vi "test_av_array_cast.vi"() -> ()   [LabVIEW 2013]
uses:
  <vilib>/userdefined/High Color/nirio_resource_hc.ctl
  <vilib>/FPGAPlugInAG/PXIe-7975R/niLvFpga_Open_PXIe-7975R.vi
  <vilib>/rvi/interface/common/dynamic/niFpgaDynamicAddResources.vi
  <vilib>/rvi/interface/common/niFpgaWaitOnOcc.vi
  <vilib>/Utility/error.llb/Error Cluster From Error Code.vi
  <vilib>/rvi/errors/niLvFpgaAdjustHostInterfaceError.vi
  <vilib>/rvi/interface/nirviOpenFPGA/nirviOpenFPGA.xnode
  FPGA Bitfiles/mixer_FPGATarget3_arraysizetest_DYaVQgTtPqo.lvbitx
  <vilib>/rvi/interface/nirviReadWriteControl/nirviReadWriteControl.xnode
  NiFpgaLv.dll
  <vilib>/rvi/interface/Simulation/niFpgaSimulationCallBeginRW.vi
panel:
  out "error out 2":errorcluster
  out "error out":errorcluster
  in  "stop":bool
  out "array 4 to 8":fxp<+/-,16,14>[](array[numeric])
  out "array 4 out":fxp<+/-,16,14>[](array[numeric])
  in  "4 in":fxp<+/-,16,14>[](array[numeric])=[0.0, 0.0, 0.0, 0.0]
  in  "4 in":bool
  in  "8 in":bool
  in  "array 8 in":fxp<+/-,16,14>[](array[numeric])=[0.0, 0.0, 0.0, 0.0, 0.0, 0.0, 0.0, 0.0]
  out "array 8 out":fxp<+/-,16,14>[](array[numeric])
  out "array 8 to 4":fxp<+/-,16,14>[](array[numeric])
  in  "resource name":T1="RIO0"
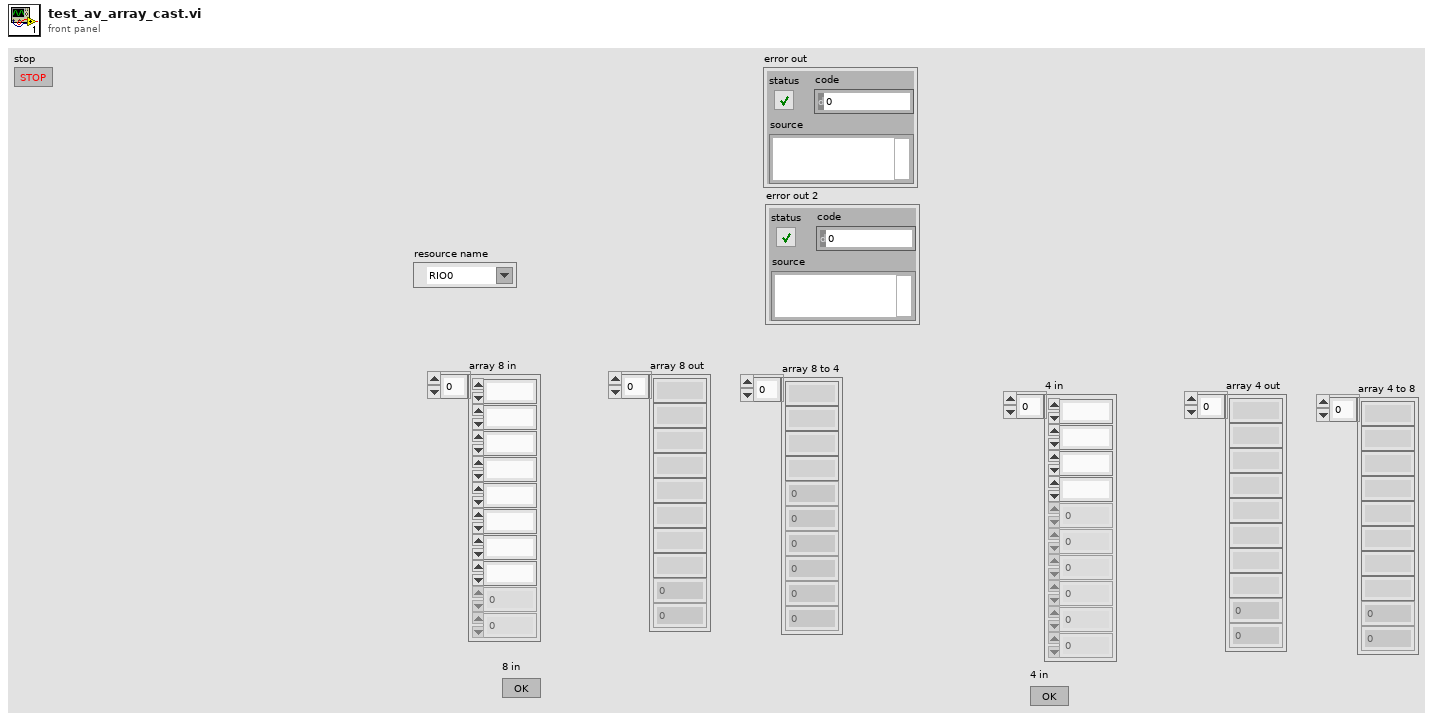
[diagram p1: front panel]
types:
  T1 = typedef "nirio_resource_hc.ctl" = tag
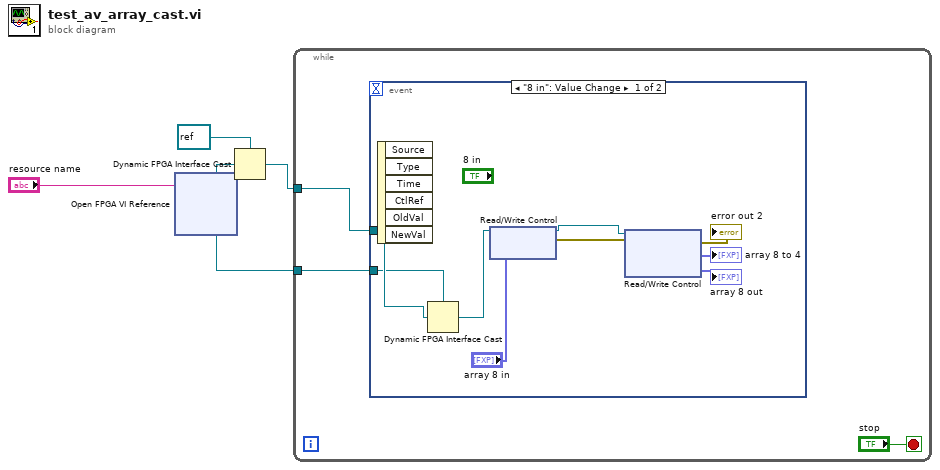
[diagram p0: block diagram]
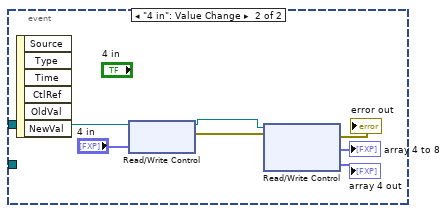
[diagram p2: hidden frame]
diagram:
  n1 = xnode "Open FPGA VI Reference"("resource name"="resource name") -> ("FPGA VI Reference Out"=w1:refnum<k20>)  [unwired: 1 in, 1 out]
  n2 = Dynamic FPGA Interface Cast(Session In=refnum<k20> refnum ("FPGA VI Reference Out"), Type=w1) -> (Session Out=w2:refnum<k20>)
  n3 = while {
    tunnel: w2 -> [w7]
    tunnel: w1 -> [w5]
    stop <- "stop" stop-if-true
    n4 = event shown="[0] \"8 in\": Value Change" {
      selector: _ -> [_ _]
      dyn-events: _ -> [_ _]
      timeout: _ -> [_ _]
      tunnel: w7 -> [w10 w23]
      tunnel: w5 -> [w9 _]
      event "8 in": Value Change {
        n5 = event-data() -> ()  [unwired: 1 in, 6 out]
        n6 = Dynamic FPGA Interface Cast(Session In=w9, Type=w10) -> (Session Out=w8:refnum<k20>)
        n7 = xnode "Read/Write Control"("FPGA VI Reference In"=w8, "array 8 in"="array 8 in") -> ("FPGA VI Reference Out"=w16:refnum<k20>, "error out"=w12:errorcluster)  [unwired: 1 in]
        n8 = xnode "Read/Write Control"("FPGA VI Reference In"=w16, "error in"=w12) -> ("error out"=→"error out 2":errorcluster, "array 8 to 4"=→"array 8 to 4":fxp<+/-,16,14>[], "array 8 out"=→"array 8 out":fxp<+/-,16,14>[])  [unwired: 1 out]
      }
      event "4 in": Value Change {
        n9 = event-data() -> ()  [unwired: 1 in, 6 out]
        n10 = xnode "Read/Write Control"("FPGA VI Reference In"=w23, "array 4 in"="4 in") -> ("FPGA VI Reference Out"=w22:refnum<k20>, "error out"=w18:errorcluster)  [unwired: 1 in]
        n11 = xnode "Read/Write Control"("FPGA VI Reference In"=w22, "error in"=w18) -> ("error out"=→"error out":errorcluster, "array 4 to 8"=→"array 4 to 8":fxp<+/-,16,14>[], "array 4 out"=→"array 4 out":fxp<+/-,16,14>[])  [unwired: 1 out]
      }
    }
  }
